vi "Extract Lines on Ramp.vi"(6 "error in":errorcluster, 9 "Image In":T1) -> (0 "error out":errorcluster, 3 "Image Out":T1, 5 "Number of Particles":i32)   [LabVIEW 2009]
uses:
  <vilib>/vision/Image Controls.llb/IMAQ Image.ctl
  <vilib>/vision/NI_Vision_Development_Module.lvlib
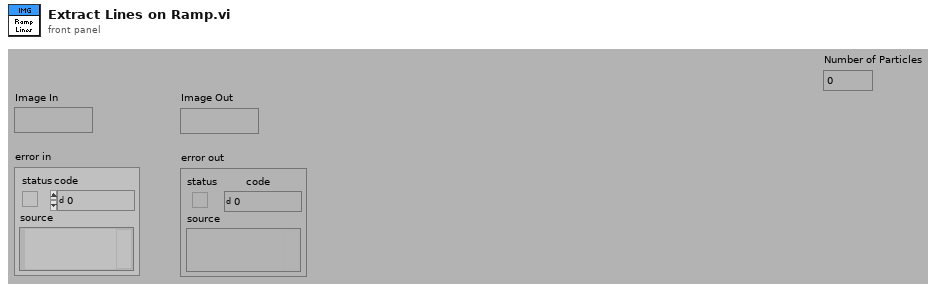
[diagram p1: front panel]
types:
  T1 = typedef "IMAQ Image.ctl" = refnum<image>
  T2 = typedef "Image Type" = u32
  T3 = cluster{"Measurement Parameter":i32, "Range Lower Value":dbl, "Range Upper Value":dbl, "Range":bool, "Measurement Type":bool}[]
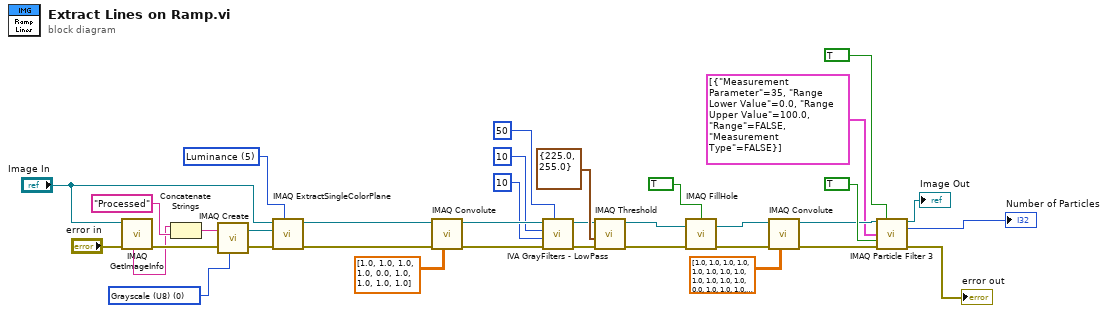
[diagram p0: block diagram]
diagram:
  w9 = T2 0 items=["Grayscale (U8)", "Grayscale (I16)", "Grayscale (SGL)", "Complex (CSG)", "RGB (U32)", "HSL (U32)", "RGB (U64)"] ("Image Type")
  w35 = 5 items=["Red", "Green", "Blue", "Hue", "Saturation", "Luminance", "Value", "Intensity"] ("Color Plane")
  n1 = call "IMAQ GetImageInfo"("error in (no error)"="error in", "Image"="Image In") -> ("error out"=w8:errorcluster, "Image Name"=w5:string)  [unwired: 8 out]
  n2 = Concatenate Strings(w5, "Processed" ("Image Name")) -> (w6:string)
  n3 = call "IMAQ Create"("Image Name"=w6, "Image Type"=w9, "error in (no error)"=w8) -> ("New Image"=w2:T1, "error out"=w3:errorcluster)  [unwired: 1 in, 1 out]
  n4 = call "IMAQ ExtractSingleColorPlane"("Color Plane"=w35, "error in (no error)"=w3, "Image Dst"=w2, "Image Src"="Image In") -> ("error out"=w34:errorcluster, "Image Dst Out"=w32:T1)  [unwired: 6 out]
  n5 = call "IMAQ Convolute"("Kernel"=sgl[][] [[1.0, 1.0, 1.0], [1.0, 0.0, 1.0], [1.0, 1.0, 1.0]], "error in (no error)"=w34, "Image Src"=w32) -> ("error out"=w31:errorcluster, "Image Dst Out"=w30:T1)  [unwired: 4 in, 3 out]
  n6 = call <vilib>:"IVA GrayFilters - LowPass.vi"("Tolerance"=50, "error in"=w31, "Filter size Y"=10, "Filter size X"=10, "Image In"=w30) -> ("error out"=w29:errorcluster, "Image Out"=w24:T1)  [unwired: 5 out]
  n7 = call "IMAQ Threshold"("error in (no error)"=w29, "Range"=cluster{"Lower value":sgl, "Upper value":sgl} {"Lower value"=225.0, "Upper value"=255.0}, "Image Src"=w24) -> ("error out"=w23:errorcluster, "Image Dst Out"=w21:T1)  [unwired: 3 in, 4 out]
  n8 = call "IMAQ FillHole"("error in (no error)"=w23, "Image Src"=w21, "Connectivity 4/8 (8)"=TRUE) -> ("error out"=w20:errorcluster, "Image Dst Out"=w18:T1)  [unwired: 1 in, 2 out]
  n9 = call "IMAQ Convolute"("Kernel"=sgl[][] [[1.0, 1.0, 1.0, 1.0, 1.0], [1.0, 1.0, 1.0, 1.0, 1.0], [1.0, 1.0, 0.0, 1.0, 1.0], [1.0, 1.0, 1.0, 1.0, 1.0], [1.0, 1.0, 1.0, 1.0, 1.0]], "error in (no error)"=w20, "Image Src"=w18) -> ("error out"=w17:errorcluster, "Image Dst Out"=w12:T1)  [unwired: 4 in, 3 out]
  n10 = call "IMAQ Particle Filter 3"("Image Src"=w12, "Connectivity 4/8 (8)"=TRUE, "Selection Values"=T3 [{"Measurement Parameter"=35, "Range Lower Value"=0.0, "Range Upper Value"=100.0, "Range"=FALSE, "Measurement Type"=FALSE}], "Keep/Remove Particles (F)"=TRUE ("Keep/Remove Particles"), "error in (no error)"=w17) -> ("Image Dst Out"=→"Image Out":T1, "Number of Particles"=→"Number of Particles":i32, "error out"=→"error out":errorcluster)  [unwired: 4 in, 4 out]
